vi "Medidas.vi"() -> ()   [LabVIEW 2024]
uses:
  <vilib>/measure/maspectr.llb/FFT Spectrum (Mag-Phase) for 1 Chan.vi
  <vilib>/measure/mascope.llb/Amplitude and Levels 1 chan.vi
  <vilib>/measure/madcrms.llb/Basic Averaged DC-RMS for 1 Chan.vi
  <vilib>/measure/NI_MAPro.lvlib
  <vilib>/Analysis/NI_AALBase.lvlib
panel:
  out "Histogram Graph":T1(graph)
  out "Magnitude":cluster{"f0":dbl, "df":dbl, "magnitude":dbl[]}(graph)
  out "RMS Values":dbl
  out "DC values":dbl
  out "Low state level":dbl
  out "High state level":dbl
  out "Amplitude":dbl
  in  "Intervals":i32
  in  "stop":bool
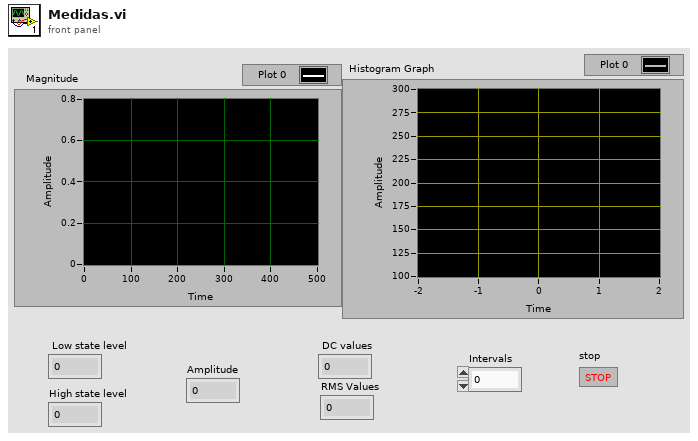
[diagram p1: front panel]
types:
  T1 = cluster{"X Values":dbl[], "Histogram: h(x)":i32[]}
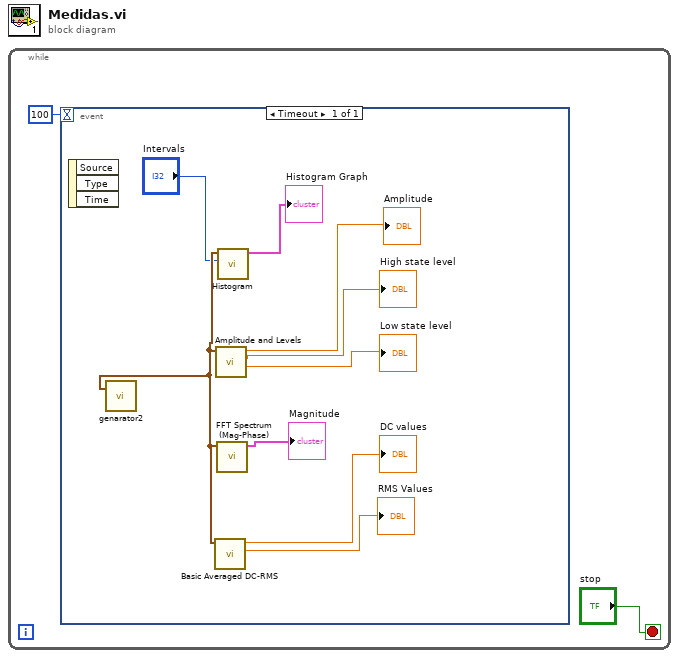
[diagram p0: block diagram]
diagram:
  n1 = while {
    stop <- "stop" stop-if-true
    n2 = event shown="[0] Timeout" {
      selector: _ -> [_]
      dyn-events: _ -> [_]
      timeout: 100 -> [_]
      event Timeout {
        n3 = event-data() -> ()  [unwired: 1 in, 3 out]
        n4 = call "genarator2.vi"() -> ("Waveform Graph 2"=w11:waveform(dbl))  [unwired: 19 in]
        n5 = call-poly <vilib>:"Basic Averaged DC-RMS.vi"("signal in"=w11) -> ("RMS value"=→"RMS Values":dbl, "DC value"=→"DC values":dbl)  [unwired: 7 in, 2 out]
        n6 = call-poly <vilib>:"Amplitude and Levels.vi"("signal in"=w11) -> ("low state level"=→"Low state level":dbl, "high state level"=→"High state level":dbl, "amplitude"=→"Amplitude":dbl)  [unwired: 7 in, 1 out]
        n7 = call-poly <vilib>:"FFT Spectrum (Mag-Phase).vi"("time signal"=w11) -> ("magnitude"=→"Magnitude":cluster{"f0":dbl, "df":dbl, "magnitude":dbl[]})  [unwired: 6 in, 4 out]
        n8 = call <vilib>:"Histogram.vi"("intervals"="Intervals", "X"=w11) -> ("Histogram Graph"=→"Histogram Graph":T1)  [unwired: 6 in, 3 out]
      }
    }
  }
